vi "File2.vi"(0 "Amplituda":dbl=1.0 format="%0.2p", 1 "Amplituda sumu":T1, 2 "Rychlost ubihani":T3=0.1 step=5e-05, 5 "Frekvence":dbl=10.0 format="%0.2p", 7 "Ubihani":bool, 9 "Offset":dbl format="%0.2p", 11 "Sirka okna (ms)":i32(listbox), 12 "Fvz":T2) -> (4 "Output":waveform(dbl)(graph), 6 "Fáze":dbl)   [LabVIEW 2019]
uses:
  Control 2.ctl
  Control 1.ctl
  Control 3.ctl
  <vilib>/measure/NI_MABase.lvlib
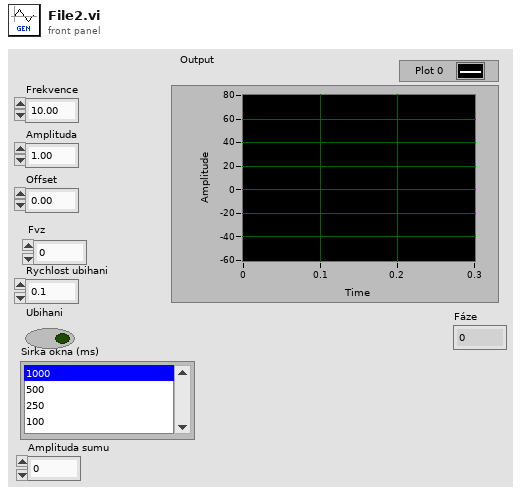
[diagram p1: front panel]
types:
  T1 = typedef "Control 3.ctl" = dbl
  T2 = typedef "Control 1.ctl" = dbl
  T3 = typedef "Control 2.ctl" = dbl
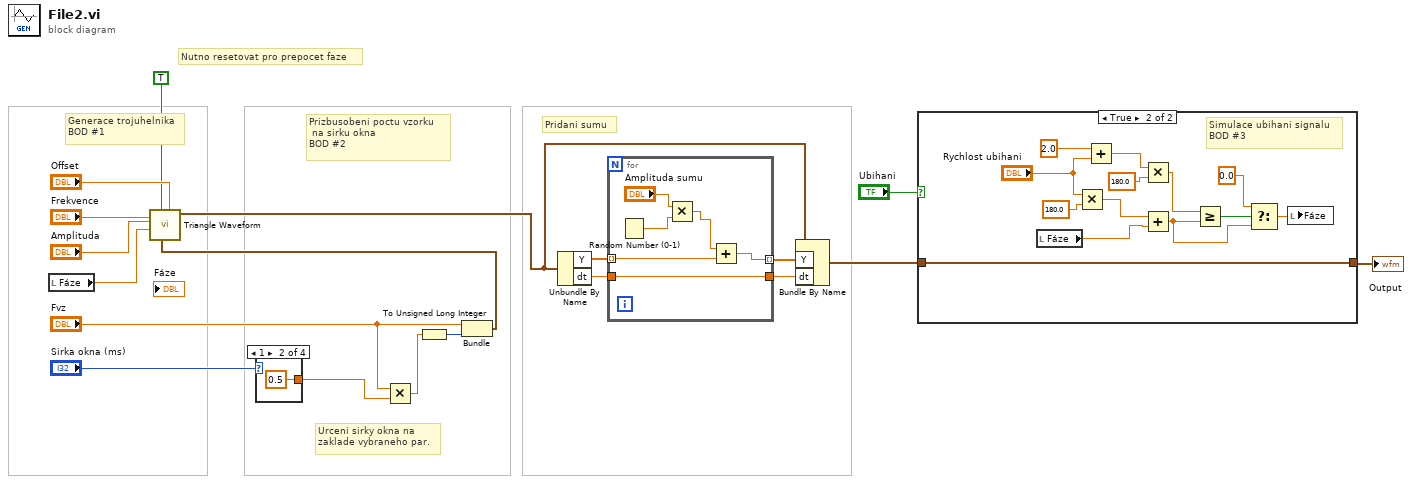
[diagram p0: block diagram]
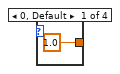
[diagram p3: hidden frame]
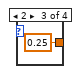
[diagram p4: hidden frame]
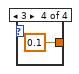
[diagram p5: hidden frame]
diagram:
  # "Pridani sumu"
  # "Nutno resetovat pro prepocet faze"
  # "Urceni sirky okna na\nzaklade vybraneho par."
  # "Prizbusobeni poctu vzorku\n na sirku okna\nBOD #2"
  # "Generace trojuhelnika\nBOD #1"
  n1 = local read "Fáze"() -> (w4:dbl)
  n2 = case shown="1" "Sirka okna (ms)" {
    tunnel: [1.0 ("X Scale.Range:Maximum") 0.5 ("X Scale.Range:Maximum") 0.25 ("X Scale.Range:Maximum") 0.1 ("X Scale.Range:Maximum")] -> w15
    frame 0, Default {
    }
    frame 1 {
    }
    frame 2 {
    }
    frame 3 {
    }
  }
  n3 = Multiply(x="Fvz", y=w15) -> (x*y=w11:T2)
  n4 = To Unsigned Long Integer(number=w11) -> (unsigned 32bit integer=w12:u32)
  n5 = Bundle("Fvz"="Fvz", w12) -> (w13:cluster{"Fvz":T2, u32})  [unwired: 1 in]
  n6 = call <vilib>:"Triangle Waveform.vi"("offset"="Offset", "sampling info"=w13, "reset signal"=TRUE, "phase"=w4, "amplitude"="Amplituda", "frequency"="Frekvence") -> ("signal out"=w5:waveform(dbl))  [unwired: 4 in, 1 out]
  n7 = Unbundle By Name(w5) -> ("Y"=w9:dbl[], "dt"=w7:dbl)
  n8 = for {
    tunnel: w9 -> [w26] mode=indexing
    tunnel: [w25] -> w8 mode=indexing
    tunnel: w7 -> [w24]
    tunnel: [w24] -> w6
    n9 = Random Number (0-1)() -> (number: 0 to 1=w28:dbl)
    n10 = Multiply(x="Amplituda sumu", y=w28) -> (x*y=w27:T1)
    n11 = Add(x=w27, y=w26) -> (x+y=w25:T1)
  }
  n12 = Bundle By Name(cluster=w5, "Y"=w8, "dt"=w6) -> (w2:waveform(dbl))
  n13 = case shown="True" "Ubihani" {
    tunnel: [w30 w32] -> w1
    tunnel: w2 -> [w30 w32]
    frame False {
    }
    frame True {
      # "Simulace ubihani signalu\nBOD #3"
      n14 = local read "Fáze"() -> (w31:dbl)
      n15 = Multiply(x="Rychlost ubihani", y=180.0 ("x")) -> (x*y=w43:T3)
      n16 = Add(x=2.0, y="Rychlost ubihani") -> (x+y=w35:T3)
      n17 = Multiply(x=w35, y=180.0 ("x")) -> (x*y=w42:T3)
      n18 = Add(x=w43, y=w31) -> (x+y=w39:T3)
      n19 = Greater Or Equal?(x=w42, y=w39) -> (x >= y?=w41:bool)
      n20 = Select(t=0.0, s=w41, f=w39) -> (s? t:f=w33:T3)
      n21 = local write "Fáze"(w33) -> ()
    }
  }
  "Output" <- w1
